vi "Remap Controls.vi"(6 "Driver Label In":T1, 7 "Manipulator Labels In":T2, 9 "Manipulator Remap":T5, 10 "Driver Remap":T4, 11 "Manipulator Diagram":T3) -> (2 "Driver Label Out":T1, 3 "Manipulator Labels out":T2)   [LabVIEW 2015]
uses:
  Common Code/Manipulator Control Remap.ctl
  Common Code/Driver Control Remap.ctl
  Common Code/Manipulator Control Label.ctl
  Common Code/Controller Diagram.ctl
  Common Code/Driver Control Label.ctl
  Common Code/Driver Control Selector.ctl
  Common Code/Manipulator Control Selector.ctl
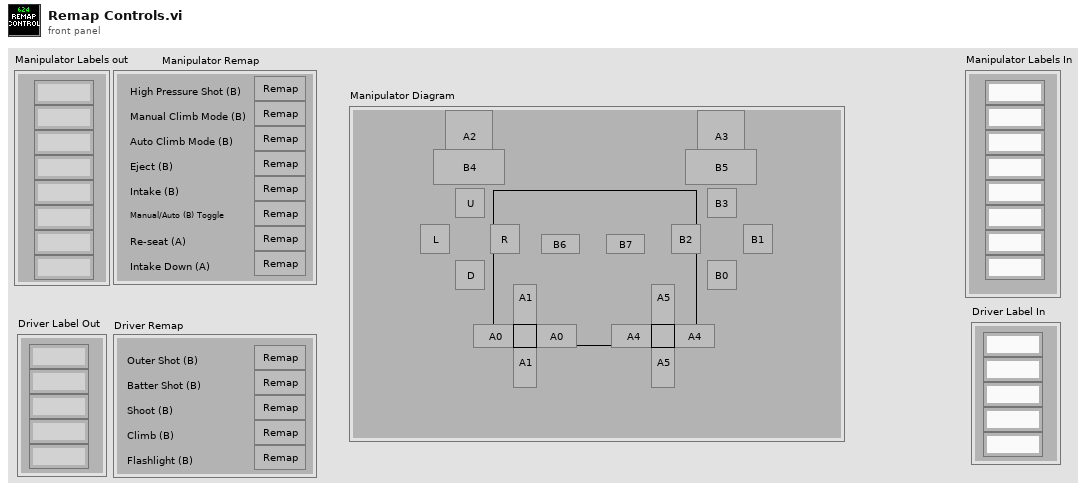
[diagram p1: front panel]
types:
  T1 = typedef "Driver Control Label.ctl" = cluster{"Outer Shot":string, "Batter Shot":string, "Shoot":string, "Climb":string, "Flashlight":string}
  T2 = typedef "Manipulator Control Label.ctl" = cluster{"High Pressure Shot":string, "Manual Climb Mode":string, "Auto Climb Mode":string, "Eject":string, "Intake":string, "Manual/Auto Toggle":string, "Re-seat":string, "Intake Down":string}
  T3 = typedef "Controller Diagram.ctl" = cluster{"Button 4":bool, "Button 5":bool, "Axis 2":bool, "Axis 3":bool, "Button 6":bool, "Button 7":bool, "Button 0":bool, "Button 1":bool, "Button 2":bool, "Button 3":bool, "POV Down":bool, "POV Right":bool, "POV Left":bool, "POV Up":bool, "Axis 1":bool, "Axis 0":bool, "Axis 4":bool, "Axis 5":bool}
  T4 = typedef "Driver Control Remap.ctl" = cluster{"Outer Shot (B)":bool, "Batter Shot (B)":bool, "Shoot (B)":bool, "Climb (B)":bool, "Flashlight (B)":bool}
  T5 = typedef "Manipulator Control Remap.ctl" = cluster{"High Pressure Shot (B)":bool, "Manual Climb Mode (B)":bool, "Auto Climb Mode (B)":bool, "Eject (B)":bool, "Intake (B)":bool, "Manual/Auto (B) Toggle":bool, "Re-seat (A)":bool, "Intake Down (A)":bool}
  T6 = typedef "Manipulator Control Selector.ctl" = enum16{"High Pressure Shot", "Manual Climb Mode", "Auto Climb Mode", "Eject", "Intake", "Manual/Auto Toggle", "Re-seat", "Intake Down", "None"}
  T7 = typedef "Driver Control Selector.ctl" = enum16{"Outer Shot", "Batter Shot", "Shoot", "Climb", "Flashlight", "None"}
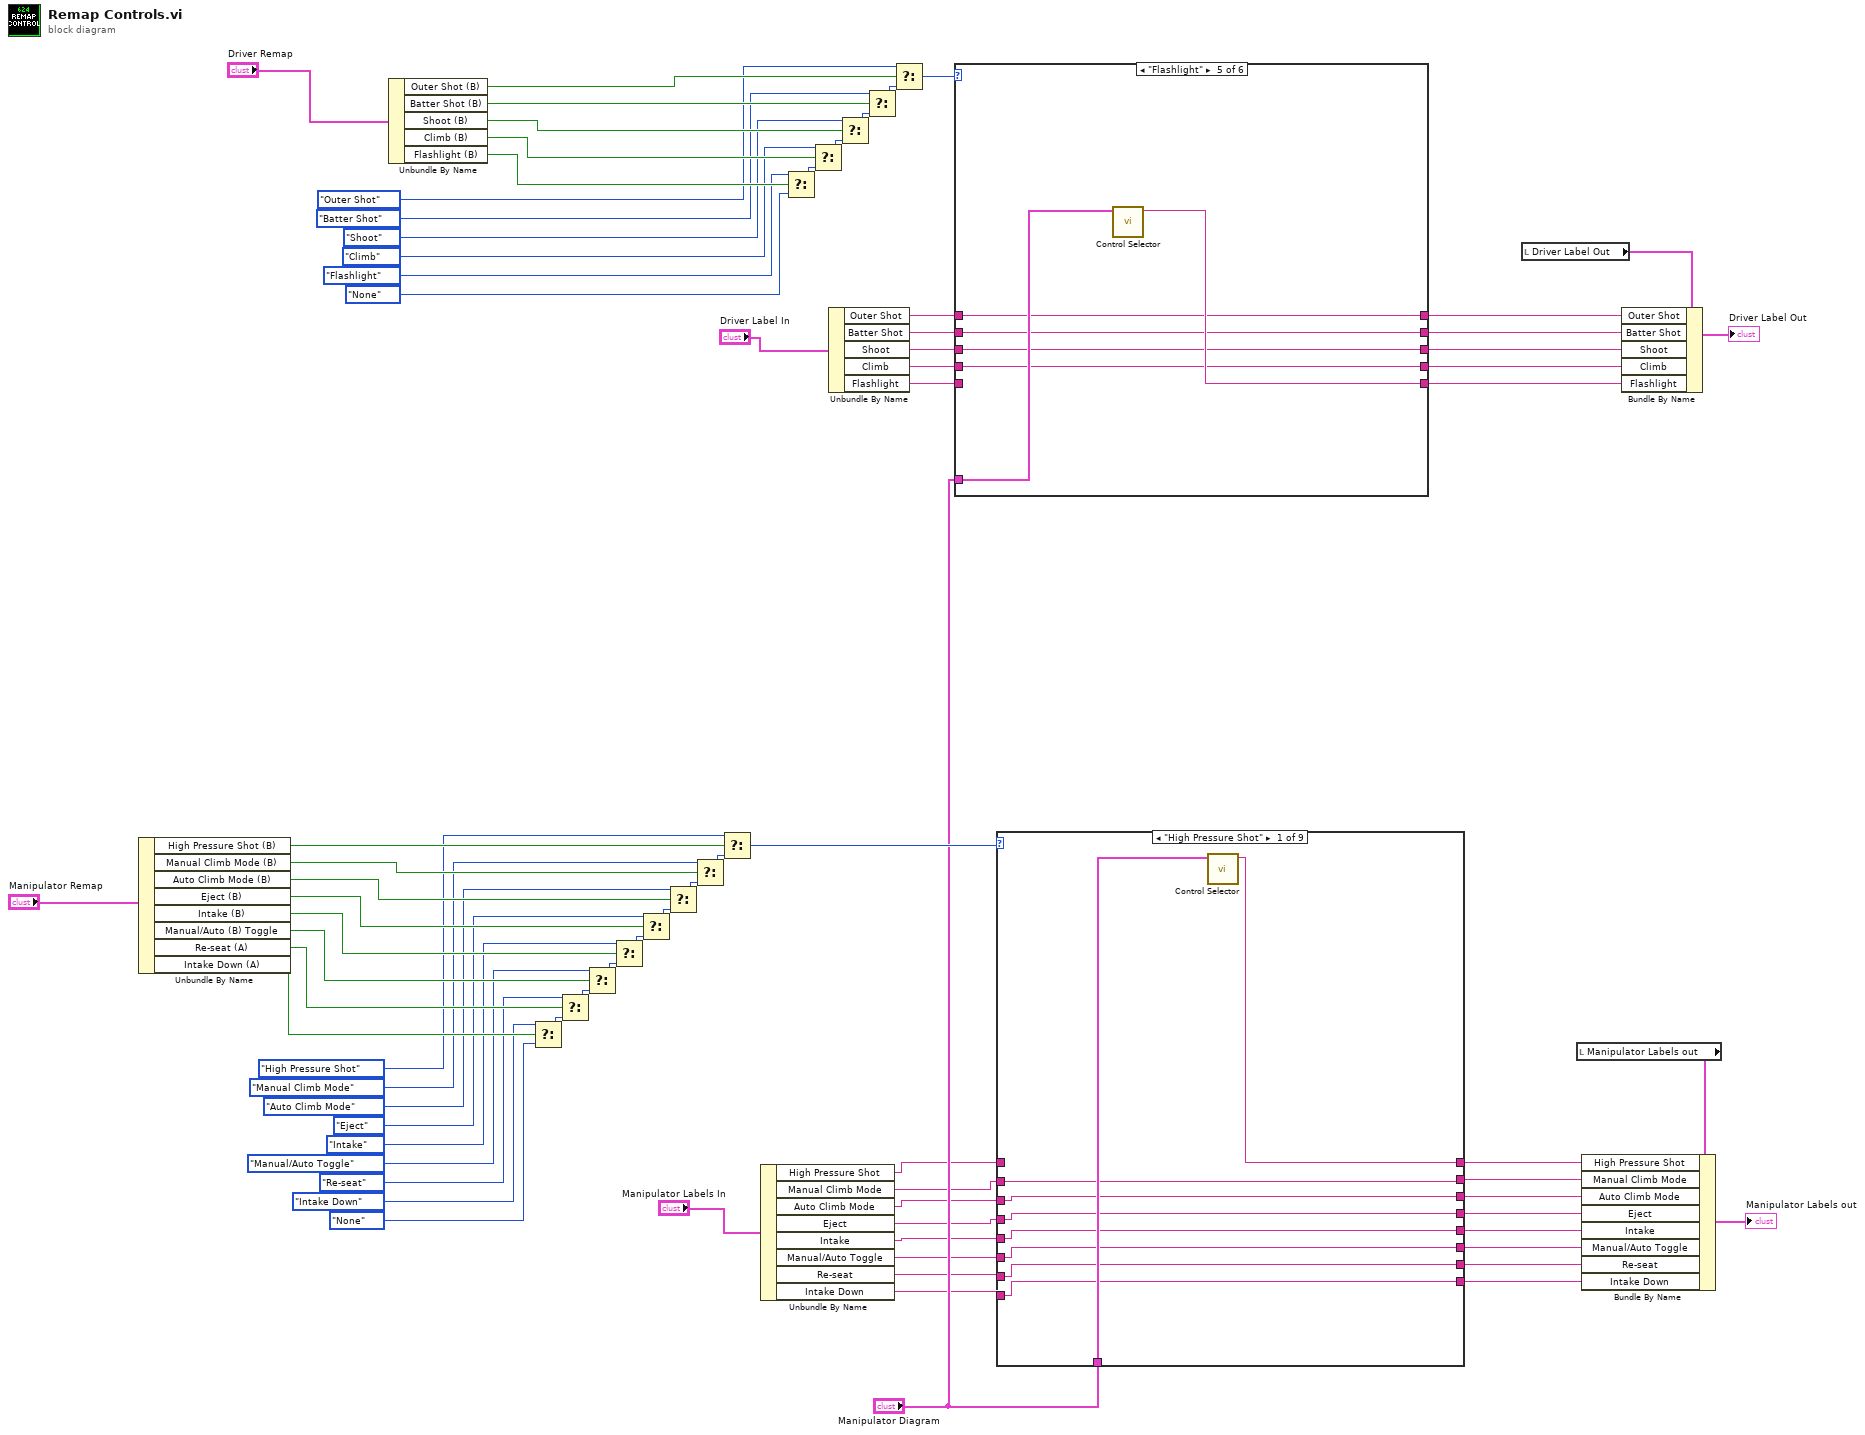
[diagram p0: block diagram]
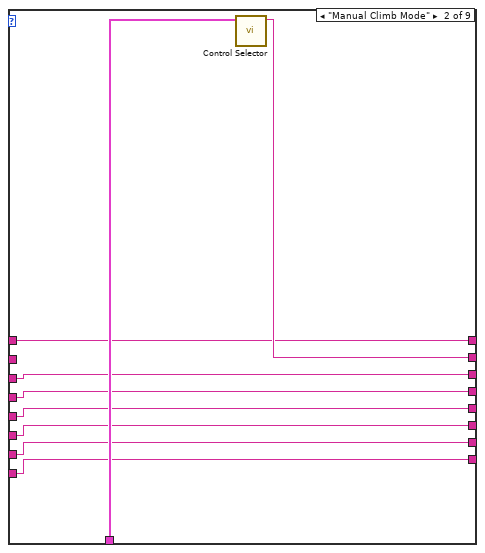
[diagram p2: hidden frame]
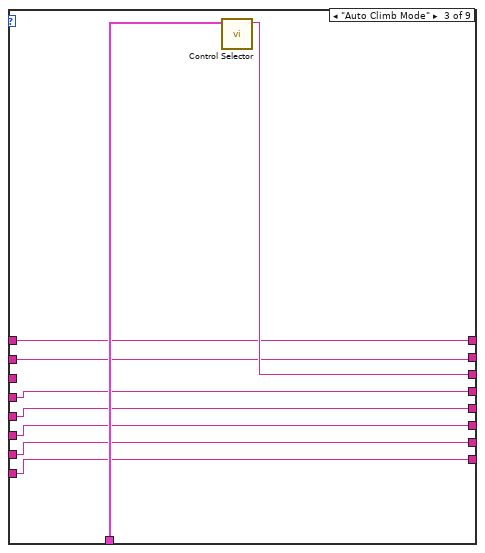
[diagram p3: hidden frame]
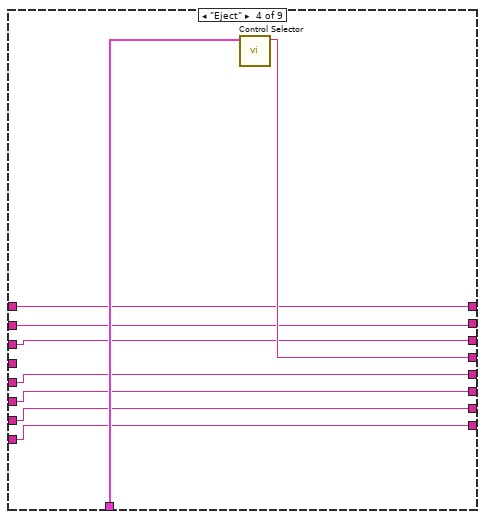
[diagram p4: hidden frame]
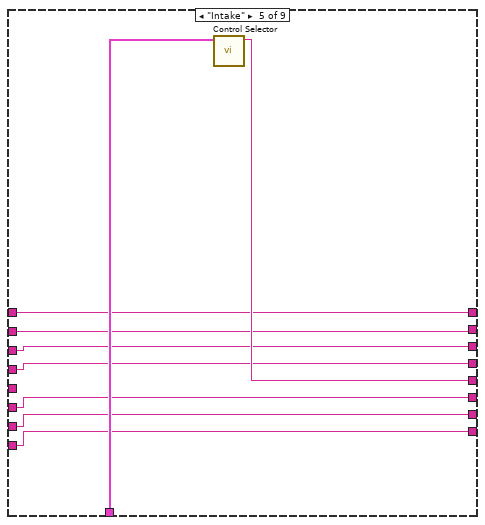
[diagram p5: hidden frame]
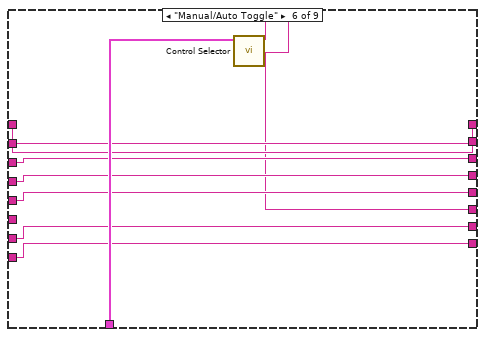
[diagram p6: hidden frame]
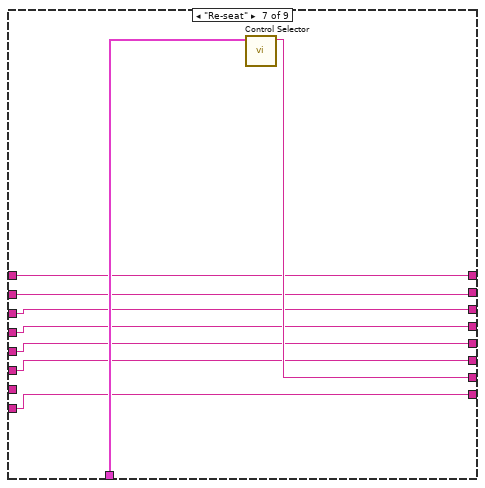
[diagram p7: hidden frame]
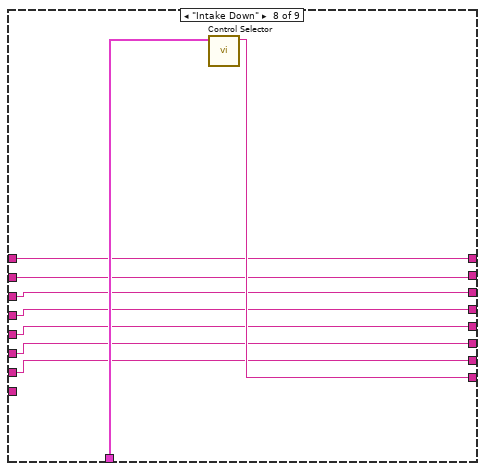
[diagram p8: hidden frame]
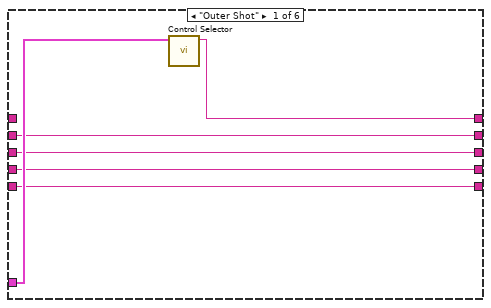
[diagram p10: hidden frame]
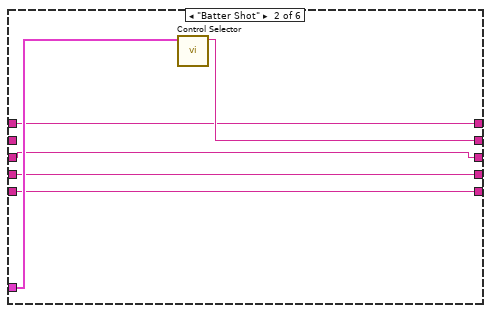
[diagram p11: hidden frame]
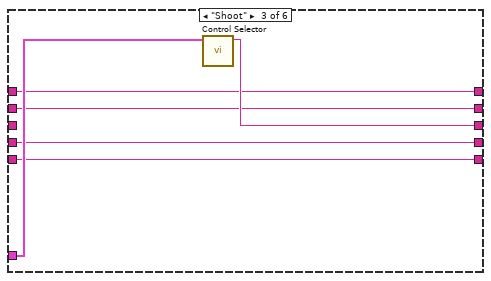
[diagram p12: hidden frame]
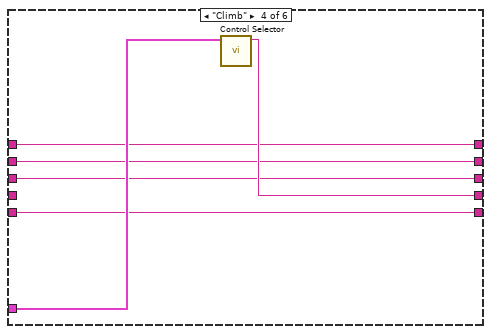
[diagram p13: hidden frame]
diagram:
  n1 = Unbundle By Name("Manipulator Remap") -> ("High Pressure Shot (B)"=w61:bool, "Manual Climb Mode (B)"=w60:bool, "Auto Climb Mode (B)"=w54:bool, "Eject (B)"=w55:bool, "Intake (B)"=w56:bool, "Manual/Auto (B) Toggle"=w57:bool, "Re-seat (A)"=w58:bool, "Intake Down (A)"=w59:bool)
  n2 = Unbundle By Name("Driver Remap") -> ("Outer Shot (B)"=w76:bool, "Batter Shot (B)"=w75:bool, "Shoot (B)"=w74:bool, "Climb (B)"=w73:bool, "Flashlight (B)"=w72:bool)
  n3 = Select(t=Manipulator_Control_Selector."Intake Down", s=w59, f=Manipulator_Control_Selector."None") -> (s? t:f=w53:T6)
  n4 = Select(t=Manipulator_Control_Selector."Re-seat", s=w58, f=w53) -> (s? t:f=w52:T6)
  n5 = Select(t=Manipulator_Control_Selector."Manual/Auto Toggle", s=w57, f=w52) -> (s? t:f=w51:T6)
  n6 = Select(t=Manipulator_Control_Selector."Intake", s=w56, f=w51) -> (s? t:f=w50:T6)
  n7 = Select(t=Manipulator_Control_Selector."Eject", s=w55, f=w50) -> (s? t:f=w49:T6)
  n8 = Select(t=Manipulator_Control_Selector."Auto Climb Mode", s=w54, f=w49) -> (s? t:f=w48:T6)
  n9 = Select(t=Manipulator_Control_Selector."Manual Climb Mode", s=w60, f=w48) -> (s? t:f=w47:T6)
  n10 = Select(t=Manipulator_Control_Selector."High Pressure Shot", s=w61, f=w47) -> (s? t:f=w37:T6)
  n11 = Unbundle By Name("Manipulator Labels In") -> ("High Pressure Shot"=w18:string, "Manual Climb Mode"=w17:string, "Auto Climb Mode"=w16:string, "Eject"=w15:string, "Intake"=w14:string, "Manual/Auto Toggle"=w13:string, "Re-seat"=w12:string, "Intake Down"=w19:string)
  n12 = Select(t=Driver_Control_Selector."Flashlight", s=w72, f=Driver_Control_Selector."None") -> (s? t:f=w68:T7)
  n13 = Select(t=Driver_Control_Selector."Climb", s=w73, f=w68) -> (s? t:f=w69:T7)
  n14 = Unbundle By Name("Driver Label In") -> ("Outer Shot"=w10:string, "Batter Shot"=w9:string, "Shoot"=w8:string, "Climb"=w7:string, "Flashlight"=w6:string)
  n15 = Select(t=Driver_Control_Selector."Shoot", s=w74, f=w69) -> (s? t:f=w70:T7)
  n16 = Select(t=Driver_Control_Selector."Batter Shot", s=w75, f=w70) -> (s? t:f=w71:T7)
  n17 = Select(t=Driver_Control_Selector."Outer Shot", s=w76, f=w71) -> (s? t:f=w23:T7)
  n18 = case shown="\"Flashlight\"" w23 {
    tunnel: "Manipulator Diagram" -> [w82 w88 w94 w99 w106 _]
    tunnel: w10 -> [_ w86 w92 w98 w101 w111]
    tunnel: w9 -> [w80 _ w91 w97 w102 w110]
    tunnel: w8 -> [w79 w85 _ w96 w103 w109]
    tunnel: w7 -> [w78 w84 w90 _ w104 w108]
    tunnel: w6 -> [w77 w83 w89 w95 _ w107]
    tunnel: [w81 w86 w92 w98 w101 w111] -> w5
    tunnel: [w80 w87 w91 w97 w102 w110] -> w4
    tunnel: [w79 w85 w93 w96 w103 w109] -> w3
    tunnel: [w78 w84 w90 w100 w104 w108] -> w2
    tunnel: [w77 w83 w89 w95 w105 w107] -> w1
    frame "Outer Shot" {
      n19 = call "Control Selector.vi"("Controller Diagram"=w82) -> ("String"=w81:string)  [unwired: 10 in]
    }
    frame "Batter Shot" {
      n20 = call "Control Selector.vi"("Controller Diagram"=w88) -> ("String"=w87:string)  [unwired: 10 in]
    }
    frame "Shoot" {
      n21 = call "Control Selector.vi"("Controller Diagram"=w94) -> ("String"=w93:string)  [unwired: 10 in]
    }
    frame "Climb" {
      n22 = call "Control Selector.vi"("Controller Diagram"=w99) -> ("String"=w100:string)  [unwired: 10 in]
    }
    frame "Flashlight" {
      n23 = call "Control Selector.vi"("Controller Diagram"=w106) -> ("String"=w105:string)  [unwired: 10 in]
    }
    frame "None" {
    }
  }
  n24 = case shown="\"High Pressure Shot\"" w37 {
    tunnel: "Manipulator Diagram" -> [w120 w129 w138 w147 w156 w165 w174 w183 _]
    tunnel: [w119 w127 w136 w145 w154 w164 w172 w181 w191] -> w32
    tunnel: [w118 w128 w135 w144 w153 w163 w171 w180 w190] -> w31
    tunnel: [w117 w126 w137 w143 w152 w162 w170 w179 w189] -> w30
    tunnel: [w116 w125 w134 w146 w151 w161 w169 w178 w188] -> w29
    tunnel: [w115 w124 w133 w142 w155 w160 w168 w177 w187] -> w28
    tunnel: [w114 w123 w132 w141 w150 w157 w167 w176 w186] -> w27
    tunnel: [w113 w122 w131 w140 w149 w159 w173 w175 w185] -> w26
    tunnel: [w112 w121 w130 w139 w148 w158 w166 w182 w184] -> w25
    tunnel: w18 -> [_ w127 w136 w145 w154 w164 w172 w181 w191]
    tunnel: w17 -> [w118 _ w135 w144 w153 w163 w171 w180 w190]
    tunnel: w16 -> [w117 w126 _ w143 w152 w162 w170 w179 w189]
    tunnel: w15 -> [w116 w125 w134 _ w151 w161 w169 w178 w188]
    tunnel: w14 -> [w115 w124 w133 w142 _ w160 w168 w177 w187]
    tunnel: w13 -> [w114 w123 w132 w141 w150 _ w167 w176 w186]
    tunnel: w12 -> [w113 w122 w131 w140 w149 w159 _ w175 w185]
    tunnel: w19 -> [w112 w121 w130 w139 w148 w158 w166 _ w184]
    frame "High Pressure Shot" {
      n25 = call "Control Selector.vi"("Controller Diagram"=w120) -> ("String"=w119:string)  [unwired: 10 in]
    }
    frame "Manual Climb Mode" {
      n26 = call "Control Selector.vi"("Controller Diagram"=w129) -> ("String"=w128:string)  [unwired: 10 in]
    }
    frame "Auto Climb Mode" {
      n27 = call "Control Selector.vi"("Controller Diagram"=w138) -> ("String"=w137:string)  [unwired: 10 in]
    }
    frame "Eject" {
      n28 = call "Control Selector.vi"("Controller Diagram"=w147) -> ("String"=w146:string)  [unwired: 10 in]
    }
    frame "Intake" {
      n29 = call "Control Selector.vi"("Controller Diagram"=w156) -> ("String"=w155:string)  [unwired: 10 in]
    }
    frame "Manual/Auto Toggle" {
      n30 = call "Control Selector.vi"("Controller Diagram"=w165) -> ("String"=w157:string)  [unwired: 10 in]
    }
    frame "Re-seat" {
      n31 = call "Control Selector.vi"("Controller Diagram"=w174) -> ("String"=w173:string)  [unwired: 10 in]
    }
    frame "Intake Down" {
      n32 = call "Control Selector.vi"("Controller Diagram"=w183) -> ("String"=w182:string)  [unwired: 10 in]
    }
    frame "None", Default {
    }
  }
  n33 = local read "Driver Label Out"() -> (w21:T1)
  n34 = local read "Manipulator Labels out"() -> (w34:T2)
  n35 = Bundle By Name(cluster=w34, "High Pressure Shot"=w32, "Manual Climb Mode"=w31, "Auto Climb Mode"=w30, "Eject"=w29, "Intake"=w28, "Manual/Auto Toggle"=w27, "Re-seat"=w26, "Intake Down"=w25) -> (→"Manipulator Labels out":T2)
  n36 = Bundle By Name(cluster=w21, "Outer Shot"=w5, "Batter Shot"=w4, "Shoot"=w3, "Climb"=w2, "Flashlight"=w1) -> (→"Driver Label Out":T1)
